vi "LS4 LoadConfigSD.vi"(1 "FileName":string) -> (0 "Command executed":bool)   [LabVIEW 2015]
doc: "Loads all LStep parameters (interface, axis parameters, controller..) from an INI-file. The format is compatible to the Wincom4-INI-file (Wincom4.ini)."
uses:
  DLL/LStep4.dll
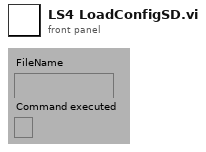
[diagram p1: front panel]
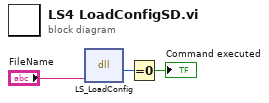
[diagram p0: block diagram]
diagram:
  n1 = dll-call lib="G:/SD/TRANCON/DLL/LStep4.dll" fn="LS_LoadConfig"("FileName"="FileName") -> ("type de retour"=w1:i32)  [unwired: 4 in, 2 out]
  n2 = Equal To 0?(x=w1) -> (x = 0?=→"Command executed":bool)
